vi "Getall_extension_numbers_response.vi"(8 "error in (no error)":errorcluster, 11 "OneOfTemplate in":refnum<class "grpc_reflection_v1alpha_ServerReflectionResponse_message_response.lvclass">) -> (0 "error out":errorcluster, 2 "Get_Val":T1, 3 "OneOfTemplate out":refnum<class "grpc_reflection_v1alpha_ServerReflectionResponse_message_response.lvclass">)   [LabVIEW 2019, in "reflection_server.lvlib" / "grpc_reflection_v1alpha_ServerReflectionResponse_message_response.lvclass"]
uses:
  grpc_reflection_v1alpha_ServerReflectionResponse_message_response.lvclass
  grpc_reflection_v1alpha_ExtensionNumberResponse.ctl
  grpc_reflection_v1alpha_ServerReflectionResponse_message_response.lvclass/grpc_reflection_v1alpha_ServerReflectionResponse_message_response.ctl
  reflection_server.lvlib
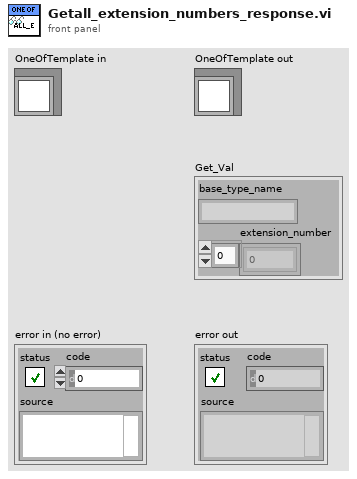
[diagram p1: front panel]
types:
  T1 = typedef "reflection_server.lvlib/grpc_reflection_v1alpha_ExtensionNumberResponse.ctl" = cluster{"base_type_name":string, "extension_number":i32[]}
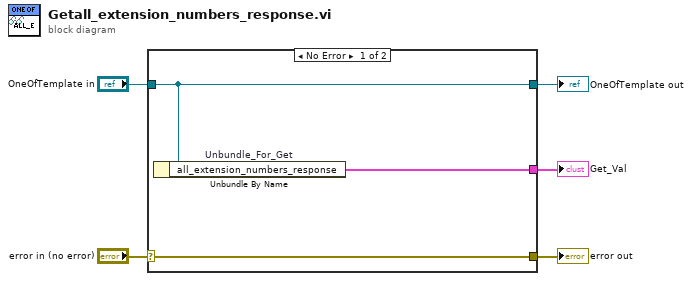
[diagram p0: block diagram]
diagram:
  n1 = case shown="No Error" "error in (no error)" {
    selector: "error in (no error)" -> [w8 w9]
    tunnel: [w8 w9] -> w4
    tunnel: [w7 w10] -> w2
    tunnel: "OneOfTemplate in" -> [w7 w10]
    tunnel: [w6 _] -> w1
    frame No Error {
      n2 = Unbundle By Name "Unbundle_For_Get"(w7) -> ("all_extension_numbers_response"=w6:T1)
    }
    frame Error {
    }
  }
  "error out" <- w4
  "OneOfTemplate out" <- w2
  "Get_Val" <- w1
